vi "Turn off All.vi"(8 "error in":errorcluster, 11 "3300 in":refnum<class "3300.lvclass">) -> (0 "error out":errorcluster, 3 "3300 out":refnum<class "3300.lvclass">)   [LabVIEW 2019, in "3300.lvlib" / "3300.lvclass"]
uses:
  Library/3300.lvclass
  C:/Users/Public/Documents/Development/builds/Instruments/Electronic Load.lvlibp/Library/Electronic Load.lvclass
  builds/Instruments/Electronic Load.lvlibp/Accessors/Read Available Channels.vi
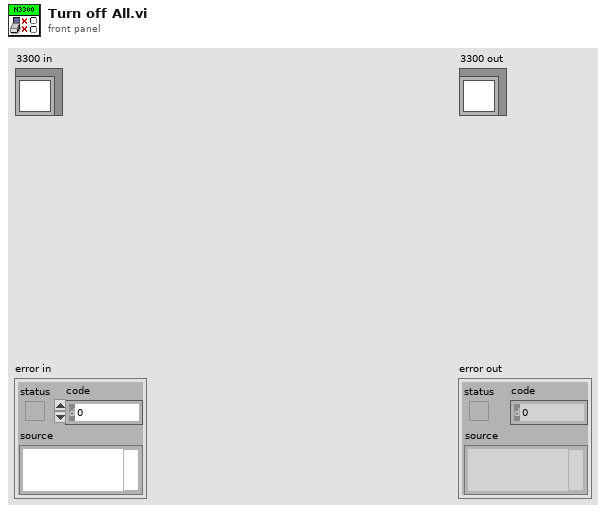
[diagram p1: front panel]
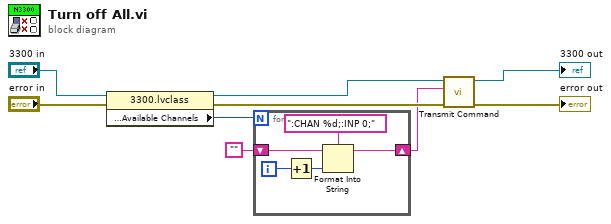
[diagram p0: block diagram]
diagram:
  n1 = property class="3300.lvclass"(reference="3300 in", error in="error in") -> (reference out=w6:refnum<class "3300.lvclass">, error out=w5:errorcluster, "Accessors:Configuration:Available Channels"=w1:i32)
  n2 = for {
    N: w1 -> [_]
    shift-right: [w13] -> w4
    shift-left: "" -> [w14]
    i -> [w10]
    n3 = Increment(x=w10) -> (x+1=w11:i32)
    n4 = Format Into String(format string=":CHAN %d;:INP 0;", initial string=w14, w11) -> (resulting string=w13:string)  [unwired: 1 in, 1 out]
  }
  n5 = call "Transmit Command.vi"("error in"=w5, "Command"=w4, "3300 in"=w6) -> ("error out"=→"error out":errorcluster, "3300 out"=→"3300 out":refnum<class "3300.lvclass">)  [unwired: 7 in]
